vi "ctrlManualForce.vi"() -> (0 "u_2":dbl, 1 "u_1":dbl, 2 "u_0":dbl, 5 "stopManualForce_DSH":bool)   [LabVIEW 2014]
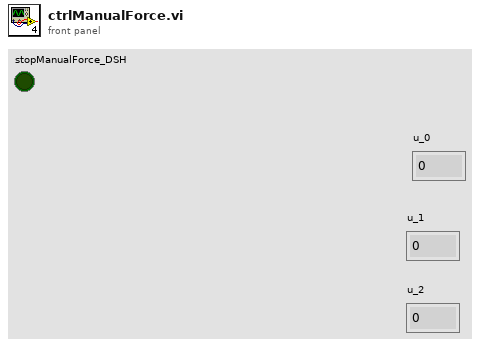
[diagram p1: front panel]
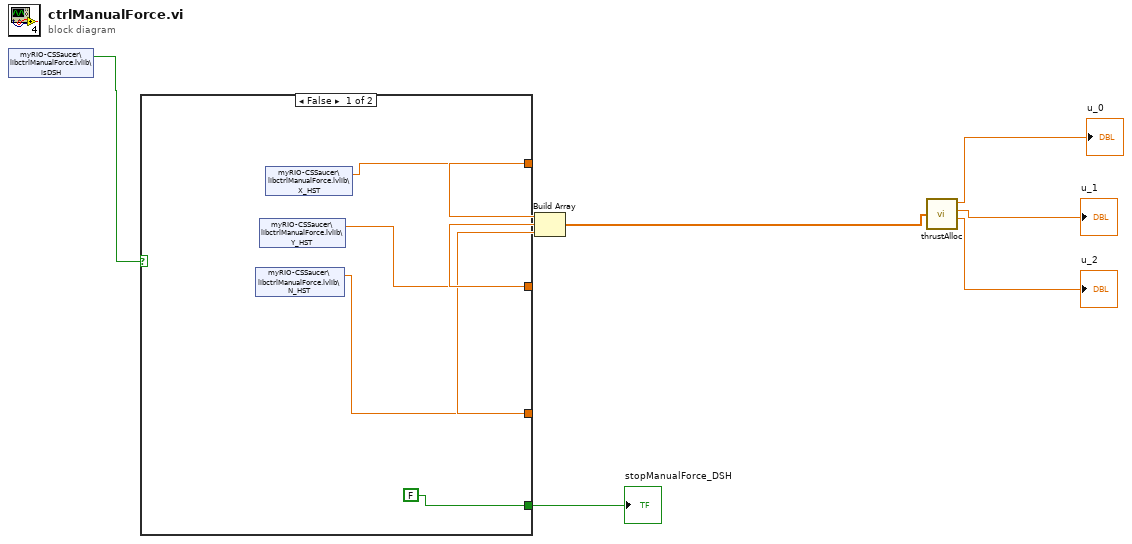
[diagram p0: block diagram]
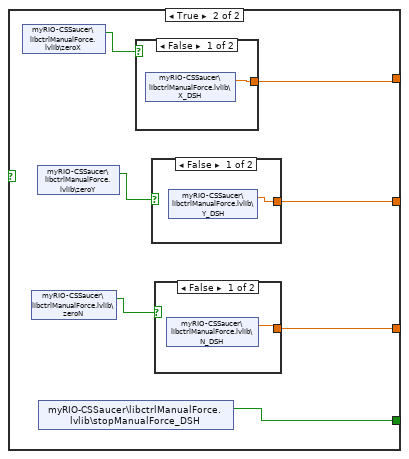
[diagram p2: hidden frame]
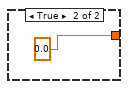
[diagram p3: hidden frame]
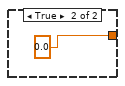
[diagram p4: hidden frame]
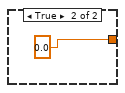
[diagram p5: hidden frame]
diagram:
  n1 = shared-variable "myRIO-CSSaucer\\libctrlManualForce.lvlib\\isDSH"() -> (w9:bool)  [unwired: 1 in, 1 out]
  n2 = case shown="False" w9 {
    tunnel: [w12 w20] -> w8
    tunnel: [w11 w18] -> w7
    tunnel: [w13 w19] -> w6
    tunnel: [FALSE w14] -> w1
    frame False {
      n3 = shared-variable "myRIO-CSSaucer\\libctrlManualForce.lvlib\\N_HST"() -> (w13:dbl)  [unwired: 1 in, 1 out]
      n4 = shared-variable "myRIO-CSSaucer\\libctrlManualForce.lvlib\\Y_HST"() -> (w11:dbl)  [unwired: 1 in, 1 out]
      n5 = shared-variable "myRIO-CSSaucer\\libctrlManualForce.lvlib\\X_HST"() -> (w12:dbl)  [unwired: 1 in, 1 out]
    }
    frame True {
      n6 = shared-variable "myRIO-CSSaucer\\libctrlManualForce.lvlib\\zeroX"() -> (w17:bool)  [unwired: 1 in, 1 out]
      n7 = shared-variable "myRIO-CSSaucer\\libctrlManualForce.lvlib\\zeroN"() -> (w16:bool)  [unwired: 1 in, 1 out]
      n8 = shared-variable "myRIO-CSSaucer\\libctrlManualForce.lvlib\\zeroY"() -> (w15:bool)  [unwired: 1 in, 1 out]
      n9 = shared-variable "myRIO-CSSaucer\\libctrlManualForce.lvlib\\stopManualForce_DSH"() -> (w14:bool)  [unwired: 1 in, 1 out]
      n10 = case shown="False" w17 {
        tunnel: [w25 0.0] -> w20
        frame False {
          n11 = shared-variable "myRIO-CSSaucer\\libctrlManualForce.lvlib\\X_DSH"() -> (w25:dbl)  [unwired: 1 in, 1 out]
        }
        frame True {
        }
      }
      n12 = case shown="False" w15 {
        tunnel: [w23 0.0] -> w18
        frame False {
          n13 = shared-variable "myRIO-CSSaucer\\libctrlManualForce.lvlib\\Y_DSH"() -> (w23:dbl)  [unwired: 1 in, 1 out]
        }
        frame True {
        }
      }
      n14 = case shown="False" w16 {
        tunnel: [w21 0.0] -> w19
        frame False {
          n15 = shared-variable "myRIO-CSSaucer\\libctrlManualForce.lvlib\\N_DSH"() -> (w21:dbl)  [unwired: 1 in, 1 out]
        }
        frame True {
        }
      }
    }
  }
  "stopManualForce_DSH" <- w1
  n16 = Build Array(w8, w7, w6) -> (w5:dbl[])
  n17 = call "thrustAlloc.vi"("tau"=w5) -> ("u_0"=→"u_0":dbl, "u_1"=→"u_1":dbl, "u_2"=→"u_2":dbl)  [unwired: 5 in]
